vi "U function.vi"(1 "Z input":dbl, 2 "Y input":dbl, 3 "Max Velocity":dbl) -> (0 "U":dbl)   [LabVIEW 2012]
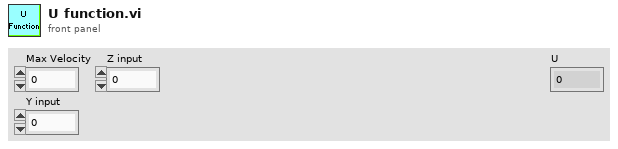
[diagram p1: front panel]
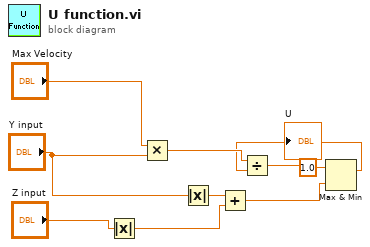
[diagram p0: block diagram]
diagram:
  n1 = Absolute Value(x="Z input") -> (abs(x)=w5:dbl)
  n2 = Multiply(x="Max Velocity", y="Y input") -> (x*y=w9:dbl)
  n3 = Absolute Value(x="Y input") -> (abs(x)=w6:dbl)
  n4 = Add(x=w6, y=w5) -> (x+y=w3:dbl)
  n5 = Max & Min(x=1.0, y=w3) -> (max(x,y)=w2:dbl)  [unwired: 1 out]
  n6 = Divide(x=w9, y=w2) -> (x/y=→"U":dbl)
